vi "Save GIF Image.vi"   [LabVIEW 2020, in "G-Image.lvlib"]
doc: "<b>This VI is polymorphic.</b>\n\nSaves an image in GIF format to disk or memory.\n\nTrue color images will be automatically quantized to 8-bit using a median-cut filter, and optional dithering. This process can be slow for large images.\n\n8-bit images are written directly to the GIF file.\n\n<b>Path In</b> can be a standard path type, or a UTF-8 encoded string."
uses:
  G-Image.lvlib
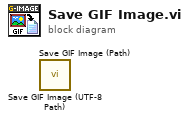
[diagram p0: block diagram]
diagram:
  n1 = call "Save GIF Image (UTF-8 Path).vi"() -> ()  [unwired: 10 in, 2 out]
  n2 = call "Save GIF Image (Path).vi"() -> ()  [unwired: 10 in, 2 out]
